vi "Check Deadband.vi"(8 "error in (no error)":errorcluster, 11 "Range Controller Actor in":refnum<class "Range Controller Actor.lvclass">) -> (0 "error out":errorcluster, 3 "Range Controller Actor out":refnum<class "Range Controller Actor.lvclass">)   [LabVIEW 2018, in "Range Controller.lvlib" / "Range Controller Actor.lvclass"]
uses:
  Range Controller Actor.lvclass
  C:/Program Files (x86)/National Instruments/LabVIEW 2018/vi.lib/ActorFramework/Actor/Actor.lvclass
  Range Controller Actor.lvclass/Range Controller Actor.ctl
  Typedefs/Deadband Result.ctl
  <vilib>/ActorFramework/Actor/Actor.lvclass/Actor.ctl
  <vilib>/ActorFramework/Message Enqueuer/Message Enqueuer.lvclass/Message Enqueuer.ctl
  <vilib>/Analysis/baseanly.llb/Mean (DBL).vi
  <vilib>/ActorFramework/Message Enqueuer/Init from Existing Queue.vi
  <vilib>/ActorFramework/Message Enqueuer/Message Enqueuer.lvclass
  <vilib>/Analysis/NI_AALBase.lvlib
  Range Controller.lvlib
  Range Controller Actor Messages/Move or Stop Range Target Msg/Move or Stop Range Target Msg.lvclass
  <vilib>/ActorFramework/Actor/Actor.lvclass
types:
  T1 = typedef "Range Controller.lvlib/Deadband Result.ctl" = enum16{"Short", "Long", "Within Tolerance"}
  T2 = typedef "MWWL Verification.lvlib/Ranges Refnum.ctl" = refnum<vi>
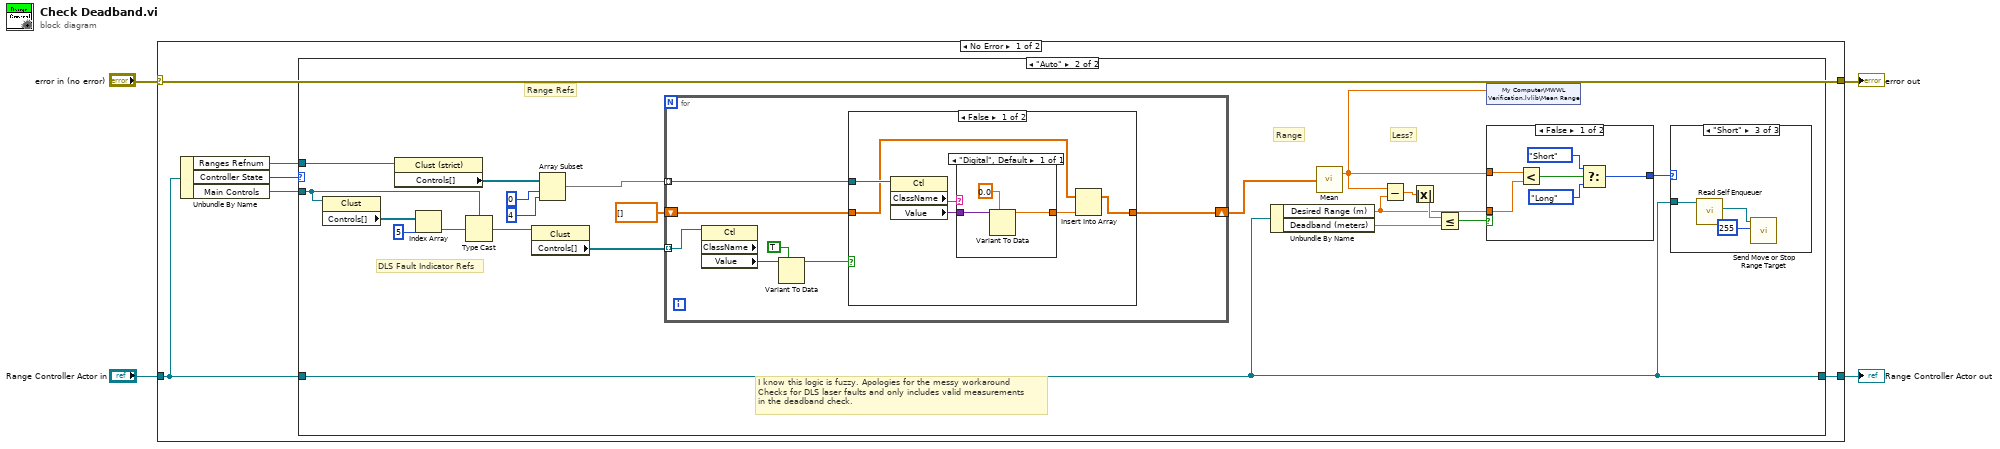
[diagram p0: block diagram]
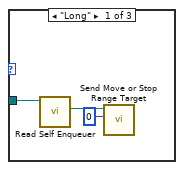
[diagram p3: hidden frame]
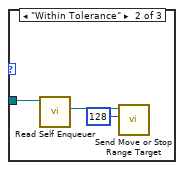
[diagram p4: hidden frame]
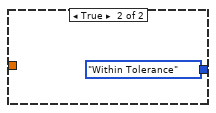
[diagram p6: hidden frame]
diagram:
  n1 = case shown="No Error" "error in (no error)" {
    selector: "error in (no error)" -> [w10 w67]
    tunnel: [w10 w67] -> w3
    tunnel: [w6 w66] -> w1
    tunnel: "Range Controller Actor in" -> [w9 w66]
    frame No Error {
      n2 = Unbundle By Name(w9) -> ("Ranges Refnum"=w8:T2, "Controller State"=w7:enum16{"Manual", "Auto"}, "Main Controls"=w5:refnum<vi>)
      n3 = case shown="\"Auto\"" w7 {
        tunnel: w9 -> [w11 w21]
        tunnel: w8 -> [_ w22]
        tunnel: [w11 w21] -> w6
        tunnel: w5 -> [_ w16]
        frame "Manual", Default {
        }
        frame "Auto" {
          # "I know this logic is fuzzy. Apologies for the messy workaround\nChecks for DLS laser faults and only includes valid measurements\nin the deadband check."
          # "Range Refs"
          # "DLS Fault Indicator Refs"
          # "Less?"
          # "Range"
          n4 = property class="Clust"(reference=w16) -> ("Controls[]"=w18:refnum<vi>[])  [unwired: 1 in, 2 out]
          n5 = property class="Clust (strict)"(reference=w22) -> ("Controls[]"=w26:refnum<vi>[])  [unwired: 1 in, 2 out]
          n6 = Index Array(array=w18, index=5) -> (element=w15:refnum<vi>)
          n7 = Type Cast(type=w16, x=w15) -> (*(type *) &x=w14:refnum<vi>)
          n8 = property class="Clust"(reference=w14) -> ("Controls[]"=w13:refnum<vi>[])  [unwired: 1 in, 2 out]
          n9 = Array Subset(array=w26, index=0, length=4 ("index")) -> (w25:refnum<vi>[])
          n10 = for {
            tunnel: w25 -> [w48] mode=indexing
            shift-right: [w43] -> w32
            shift-left: dbl[] [] -> [w44]
            tunnel: w13 -> [w42] mode=indexing
            n11 = property class="Ctl" props=["ClassName", "Value"](reference=w42) -> ("Value"=w47:variant)  [unwired: 1 in, 3 out]
            n12 = Variant To Data(type=TRUE, Variant=w47) -> (data=w45:bool)  [unwired: 1 in, 1 out]
            n13 = case shown="False" w45 {
              tunnel: w48 -> [w54 _]
              tunnel: [w49 w58] -> w43
              tunnel: w44 -> [w51 w58]
              frame False {
                n14 = property class="Ctl"(reference=w54) -> ("ClassName"=w53:string, "Value"=w52:variant)  [unwired: 1 in, 2 out]
                n15 = case shown="\"Digital\", Default" w53 {
                  tunnel: w52 -> [w57]
                  tunnel: [w55] -> w50
                  frame "Digital", Default {
                    n16 = Variant To Data(type=0.0 ("Desired Range (m)"), Variant=w57) -> (data=w55:dbl)  [unwired: 1 in, 1 out]
                  }
                }
                n17 = Insert Into Array(array=w51, new element=w50) -> (w49:dbl[])  [unwired: 1 in]
              }
              frame True {
              }
            }
          }
          n18 = Unbundle By Name(w21) -> ("Desired Range (m)"=w27:dbl, "Deadband (meters)"=w28:dbl)
          n19 = call-poly <vilib>:"Mean.vi"("X"=w32) -> ("mean"=w12:dbl)  [unwired: 1 out]
          n20 = Subtract(x=w12, y=w27) -> (x-y=w31:dbl)
          n21 = Absolute Value(x=w31) -> (abs(x)=w29:dbl)
          n22 = Less Or Equal?(x=w29, y=w28) -> (x <= y?=w30:bool)
          n23 = case shown="False" w30 {
            tunnel: w12 -> [w61 _]
            tunnel: [w62 Deadband_Result."Within Tolerance" ("Deadband Result")] -> w20
            tunnel: w27 -> [w60 _]
            frame False {
              n24 = Less?(x=w61, y=w60) -> (x < y?=w59:bool)
              n25 = Select(t=Deadband_Result."Short" ("Deadband Result"), s=w59, f=Deadband_Result."Long" ("Deadband Result")) -> (s? t:f=w62:T1)
            }
            frame True {
            }
          }
          n26 = shared-variable "My Computer\\MWWL Verification.lvlib\\Mean Range"(w12) -> ()  [unwired: 1 in, 1 out]
          n27 = case shown="\"Short\"" w20 {
            tunnel: w21 -> [w35 w38 w41]
            frame "Long" {
              n28 = call <vilib>:"Read Self Enqueuer.vi"("Actor"=w35) -> ("Self Enqueuer"=w34:refnum<class "Message Enqueuer.lvclass">)  [unwired: 10 in]
              n29 = call "Send Move or Stop Range Target.vi"("Target Speed & Direction"=i16 0, "Message Enqueuer in"=w34) -> ()  [unwired: 8 in, 2 out]
            }
            frame "Within Tolerance" {
              n30 = call <vilib>:"Read Self Enqueuer.vi"("Actor"=w38) -> ("Self Enqueuer"=w37:refnum<class "Message Enqueuer.lvclass">)  [unwired: 10 in]
              n31 = call "Send Move or Stop Range Target.vi"("Target Speed & Direction"=i16 128, "Message Enqueuer in"=w37) -> ()  [unwired: 8 in, 2 out]
            }
            frame "Short" {
              n32 = call <vilib>:"Read Self Enqueuer.vi"("Actor"=w41) -> ("Self Enqueuer"=w40:refnum<class "Message Enqueuer.lvclass">)  [unwired: 10 in]
              n33 = call "Send Move or Stop Range Target.vi"("Target Speed & Direction"=i16 255, "Message Enqueuer in"=w40) -> ()  [unwired: 8 in, 2 out]
            }
          }
        }
      }
    }
    frame Error {
    }
  }
  "error out" <- w3
  "Range Controller Actor out" <- w1
